vi "Image Acquiring Module.vi"(7 "Scan Status in":T1, 8 "Error in":errorcluster) -> (0 "Error Out":errorcluster)   [LabVIEW 2018]
uses:
  Controls/scan status.ctl
  Controls/FGV Actions.ctl
  Controls/Queue Manager Actions.ctl
  Controls/QueueNames.ctl
  Controls/MessagePacket.ctl
  Controls/Save Bline to Mem Control.ctl
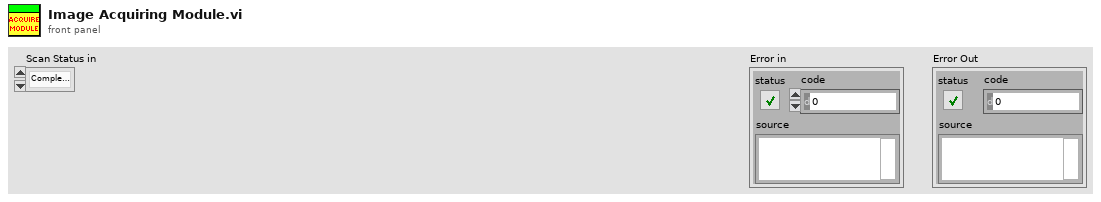
[diagram p1: front panel]
types:
  T1 = typedef "scan status.ctl" = enum16{"Complete Scan(ThorOCT)", "Complete Scan(PSOCT)", "Start(ThorOCT Spatial)", "Start(ThorOCT Spectral)", "Start(GPU FFT)", "Start(Alazar FFT)", "Scan(ThorOCT Spatial)", "Scan(ThorOCT Spectral)", "Scan(GPU FFT)", "Scan(Alazar FFT)", "Finish Scan(ThorOCT)", "Finish Scan(PSOCT)", "Scan(simulate)", "Start(ROI)"}
  T2 = typedef "FGV Actions.ctl" = enum16{"Init", "Set", "Get", "Clear"}
  T3 = typedef "System Parameters.ctl" = cluster{"Optical Parameters":T4, "Vibratome":T5, "Table Stages":T6, "Imaging Parameter":T9, "Galvo HW Parameters":cluster{"Analog Out Channel":tag, "Min Voltage":dbl, "Max Voltage":dbl, "Pixel Clock Source":tag, "Sample Rate":dbl, "Line Clock Out Ch":tag}, "Alazar parameters":T11, "Mosaic Paramter":cluster{"X Axis":cluster{"Start [mm]":dbl, "Steps [pts]":dbl, "End [mm]":dbl}, "Y Axis":cluster{"Start [mm]":dbl, "Steps [pts]":dbl, "End [mm]":dbl}, "Scan Pattern":enum16{"Uni-directional", "Bi-Directional", "Spiral Out", "Spiral In"}, "Overlap Options":cluster{"Overlap Type":enum16{"No Overlap", "X Only", "Y Only", "X and Y"}, "Percent Overlap":u8, "Justify":enum16{"Start", "Center", "End"}}}, "Manual Controls":T18, "Vibratome Axis":T21}
  T4 = typedef "Optical Parameters.ctl" = cluster{"Obj. Focal Length [mm]":dbl, "Scan Lens EFL[mm]":dbl, "Tube Lens EFL[mm]":dbl, "Galvo V Range (+/-)":dbl, "Galvo Max Half Angle [Deg]":dbl, "Max Galvo Range[%]":dbl}
  T5 = typedef "Vibratome Parameters.ctl" = cluster{"Z Bottom [mm]":dbl, "Pre Cut Dwell [s]":dbl, "Blade Frequency [RPM]":u16, "Slice Speed [mm/s]":dbl, "Post Cut Dwell [s]":dbl, "Ramp Time [s]":dbl, "Start X [mm]":dbl, "Start Y [mm]":dbl, "Slice Length [mm]":dbl, "Slice Axis":enum16{"X Axis", "Y Axis", "Z Axis"}, "Controller VISA Ref":refnum<visa-resource-name>, "Blade Frequency [Hz]":u16, "Analog Out Channel":tag, "Pixel Clock Source":tag}
  T6 = typedef "Translation Stage Parameters.ctl" = cluster{"X Stage":T7, "Y Stage":T7, "Z Stage":T7}
  T7 = typedef "Translation Stage Cluster.ctl" = cluster{"Position":dbl, "Is.Enabled?":bool, "Is.Connected?":bool, "Device SN":string, "AccelerationMaximum":dbl, "VelocityMaximum":dbl, "Acceleration":dbl, "Velocity":dbl, "waitTimeout (ms)":i32, "Model":T8, "Is.Homed?":bool}
  T8 = typedef "Translation Stage Types.ctl" = enum16{"None", "Thorlabs LTS", "Thorlabs MLJ"}
  T9 = typedef "Imaging Parameters.ctl" = cluster{"Raster Scan Direction":T10, "Pixel Dwell Time [Clock Cycles]":u16, "Flyback Time [Clock Cycles]":u16, "XY Center [um]":cluster{"X":dbl, "Y":dbl}, "Pixel Step Size [um] X":dbl, "XY Image Size":enum16{"32 x 32", "64 x 64", "128 x 128", "256 x 256", "512 x 512", "1024 x 1024", "2048 x 2048"}, "Custom":bool, "Custom Size":cluster{"X":u16, "Y":u16}, "Line Averages":u8, "Pixel Step Size [um] Y":dbl}
  T10 = typedef "Scan Direction.ctl" = enum16{"Uni Directional", "Bi Directional", "None"}
  T11 = typedef "Alazar parameters.ctl" = cluster{"Trigger Settings":cluster{"General Trigger Settings":T12, "Trigger Engine 1":T13, "Trigger Engine 2":T13}, "Device ID":T14, "Ch A Input Control":T15, "Ch B Input Control":T15, "Acq Settings":T16, "Capture Clock":T17}
  T12 = typedef "General Trigger Settings.ctl" = cluster{"Trigger Operation":u32, "Coupling ID":u32, "Range ID":u32, "Delay":u32, "Timeout Ticks":u32, "Mode":u32, "Parameter":u32}
  T13 = typedef "Trigger Engine Controls.ctl" = cluster{"Trigger Engine":u32, "Source":u32, "Slope":u32, "Level":u32}
  T14 = typedef "Alazar Device ID.ctl" = cluster{"System ID":u32, "Board ID":u32}
  T15 = typedef "Channel Input Controls.ctl" = cluster{"Channel":u8, "Coupling":u32, "Range":u32, "Impedance":u32}
  T16 = typedef "Alazar Acquisition Settings.ctl" = cluster{"Record Length":u32, "Offset":u32, "Records Per Buffer":u32, "Records Count (Records/Acq)":u32, "Window Type":u32, "Footer":u32, "Samples per record":u32, "Output Format":u32}
  T17 = typedef "Clock Controls.ctl" = cluster{"Sample Rate":u32, "Decimation":u32, "Source":u32, "Edge":u32}
  T18 = typedef "Manual Controls.ctl" = cluster{"Z0":dbl, "First image height":dbl, "Data Path":path, "Save parameters":T19, "Center Galvos":bool, "Acquisition mode":T20, "PSOCT Channel":u32, "Save":bool, "AIP rotation angle":dbl, "Scan Parameters":cluster{"# Scan":cluster{"#Ascan":i32, "#Bscan":i32}, "# Rpt":cluster{"#ARpt":i32, "#BRpt":i32}, "Aline Rate":u16, "# Extra":cluster{"# ARpt_extra":i32, "#Brtn_extra":i32}}, "ROI Parameters":cluster{"ROI (mm)":cluster{"X (mm)":dbl, "Y (mm)":dbl}, "Shift (mm)":cluster{"Xshift (mm)":sgl, "Yshift (mm)":sgl}}, "Objective":u16, "auto adjust focus":bool, "ret ds":bool, "Pause?":bool}
  T19 = typedef "FFT parameters.ctl" = cluster{"start pixel":i32, "#pixels to save":i32}
  T20 = typedef "FFT mode.ctl" = enum16{"ThorOCT B line", "ThorOCT Spectral", "ThorOCT FFT", "Alazar B line", "Alazar FFT", "GPU FFT", "Alazar Spectral", "Simulation", "auto adjust focus"}
  T21 = typedef "Vibratome Param.ctl" = cluster{"Start [mm](first cut height)":dbl, "slice thickness[um]":dbl, "#slice":u16, "slice thick2[um]":dbl, "#thin slices":u16, "image thickness(um)":dbl, "#images":u16, "image depth2":dbl, "#image depth2":u16}
  T22 = enum16{"Init", "Configure", "Configure Data", "Generate Scan Pattern", "Start Acquire Raw", "Start Acquire Data", "Acquire RAW", "Acquire Data", "Stop Acquire", "Uninit"}
  T23 = typedef "Save Bline to Mem Control.ctl" = enum16{"Output data", "Save(ThorOCT)", "Save(PSOCT)", "FFT and Save", "Uninit", "PSOCT Spectral buffer Set", "PSOCT Spatial buffer Set", "PSOCT Spectral buffer Init", "PSOCT Spatial buffer Init", "ThorOCT Spectral buffer Init", "ThorOCT Spatial buffer Init", "ThorOCT Spectral buffer Set", "ThorOCT Spatial buffer Set", "ThorOCT Spectral Save", "Alazar Spectral Save"}
  T24 = typedef "MessagePacket.ctl" = cluster{"Message":string, "Parameter":variant}
  T25 = typedef "QueueNames.ctl" = enum16{"Main GUI", "Main Scan Processor", "Main Processing", "Main Saving", "Main Display", "Main Table Stage GUI", "Main Table Stage Proc.", "Scan Engine", "Vibratome GUI", "Vibratome Processor", "Slice Engine"}
  T26 = typedef "Queue Manager Actions.ctl" = enum16{"Init", "Enqueue", "Enqueue All", "Preview Queue", "Dequeue", "Get Status", "Flush Queue", "Flush All Queues", "Release All Queues", "Release Queue", "Enqueue at Opposite End"}
  T27 = cluster{"# Scan":cluster{"#Ascan":i32, "#Bscan":i32}, "# Rpt":cluster{"#ARpt":i32, "#BRpt":i32}, "Aline Rate":u16, "# Extra":cluster{"# ARpt_extra":i32, "#Brtn_extra":i32}}
  T28 = cluster{"ROI (mm)":cluster{"X (mm)":dbl, "Y (mm)":dbl}, "Shift (mm)":cluster{"Xshift (mm)":sgl, "Yshift (mm)":sgl}}
  T29 = typedef "ScanType.ctl" = enum16{"Single Frame", "Continuous Frame", "ROI Line", "Vibratome", "Mosaic", "Mosaic + Slice"}
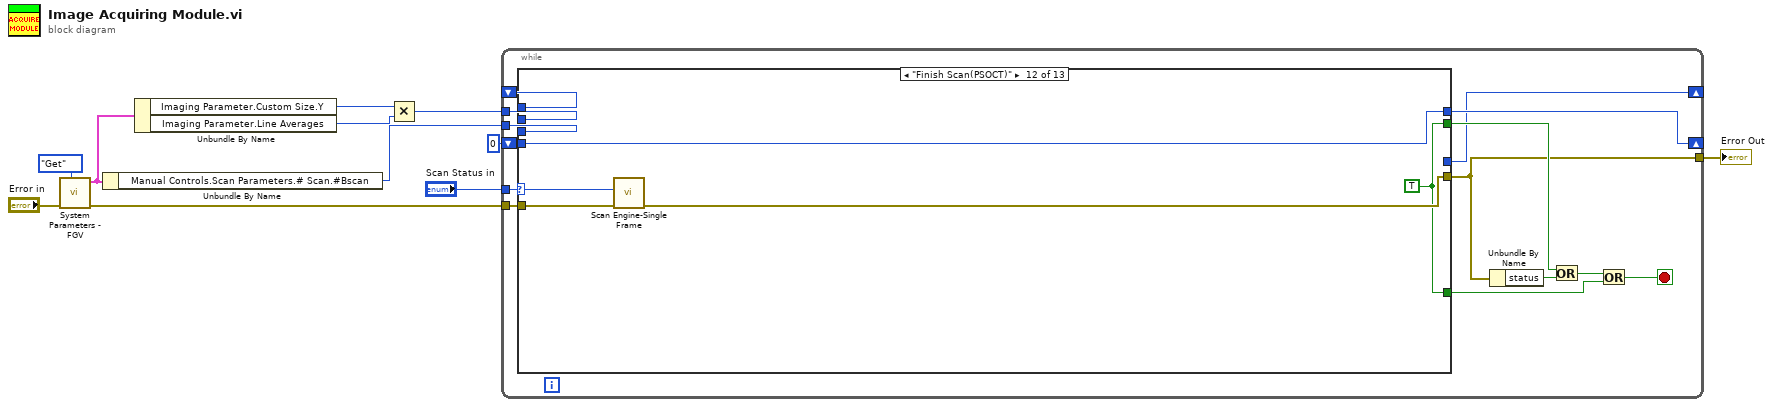
[diagram p0: block diagram]
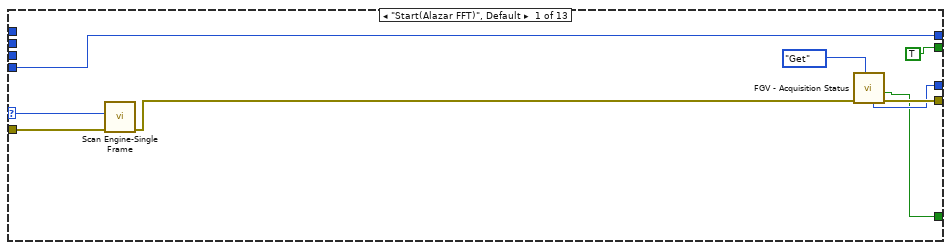
[diagram p2: hidden frame]
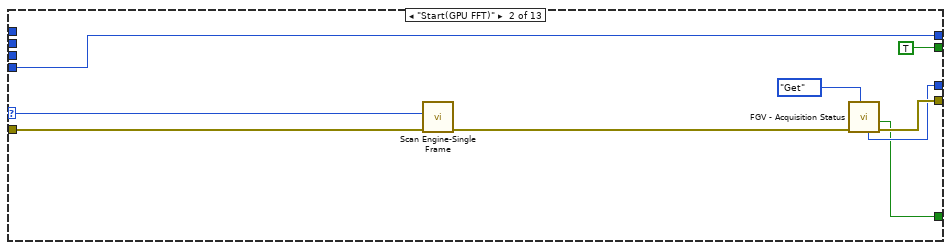
[diagram p3: hidden frame]
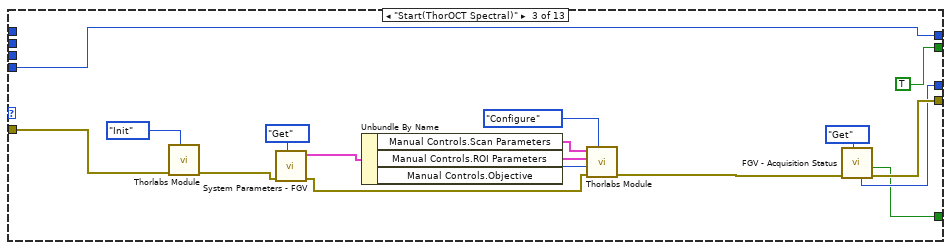
[diagram p4: hidden frame]
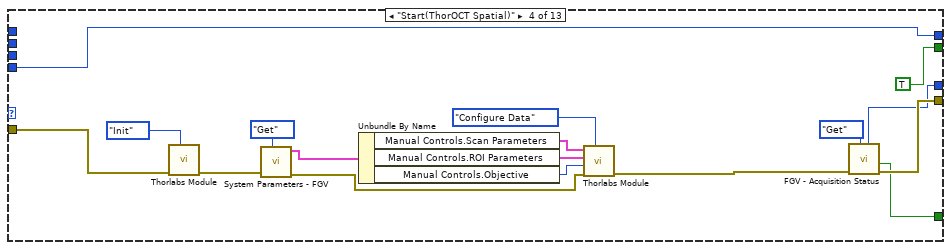
[diagram p5: hidden frame]
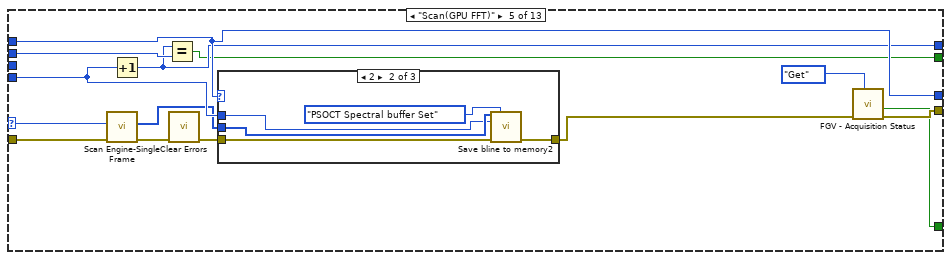
[diagram p6: hidden frame]
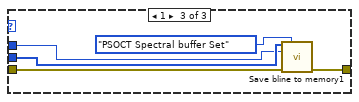
[diagram p8: hidden frame]
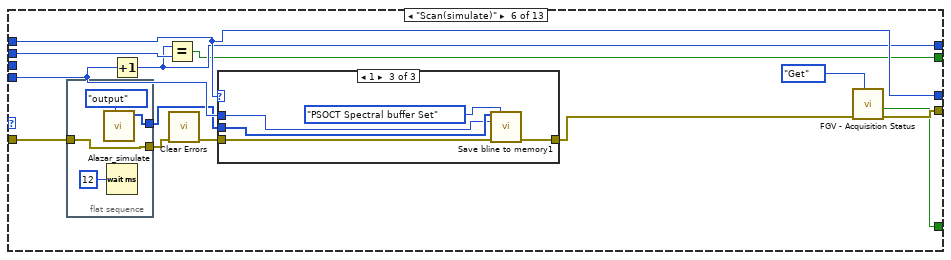
[diagram p9: hidden frame]
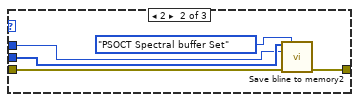
[diagram p11: hidden frame]
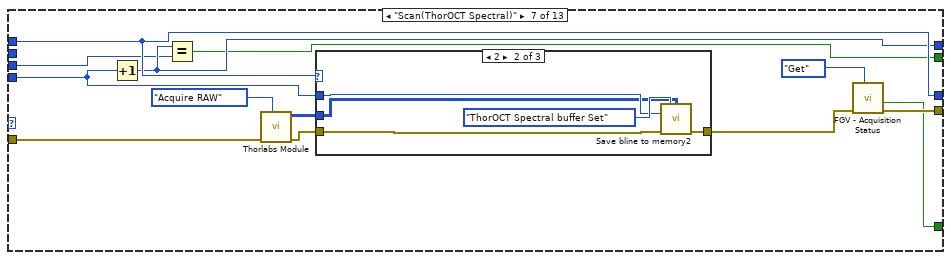
[diagram p12: hidden frame]
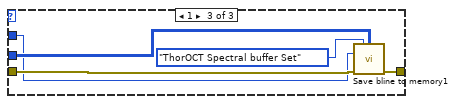
[diagram p14: hidden frame]
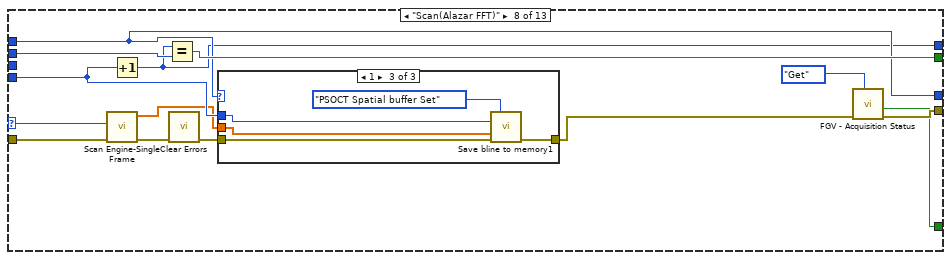
[diagram p15: hidden frame]
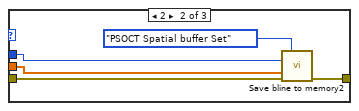
[diagram p17: hidden frame]
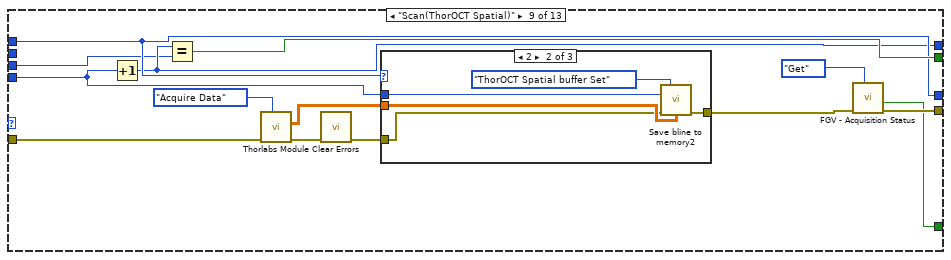
[diagram p18: hidden frame]
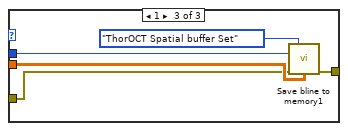
[diagram p20: hidden frame]
diagram:
  n1 = call "System Parameters - FGV.vi"("Actions"=FGV_Actions."Get", "Error In"="Error in") -> ("Error Out"=w2:errorcluster, "System Parameters [Out]"=w3:T3)  [unwired: 8 in]
  n2 = Unbundle By Name(w3) -> ("Manual Controls.Scan Parameters.# Scan.#Bscan"=w5:i32)
  n3 = Unbundle By Name(w3) -> ("Imaging Parameter.Custom Size.Y"=w8:u16, "Imaging Parameter.Line Averages"=w7:u8)
  n4 = Multiply(x=w8, y=w7) -> (x*y=w6:u16)
  n5 = while {
    tunnel: w2 -> [w23]
    tunnel: "Scan Status in" -> [w25]
    shift-right: [w24] -> _
    shift-left: u32 0 ("bline count") -> [w21]
    tunnel: w6 -> [w18]
    shift-right: [w16] -> _
    shift-left: _ -> [w17]
    tunnel: [w15] -> w9
    tunnel: w5 -> [w12]
    stop <- w19 stop-if-true
    n6 = case shown="\"Finish Scan(PSOCT)\"" w25 {
      selector: w25 -> [w31 w41 _ _ w85 _ _ w167 _ _ _ w246 _]
      tunnel: w23 -> [w34 w43 w54 w71 w86 w104 w135 w168 w184 w213 w226 w249 w252]
      tunnel: [w28 w37 w57 w74 w81 w108 w137 w159 w187 w208 w230 w247 w250] -> w15
      tunnel: [TRUE TRUE TRUE TRUE w87 w111 w140 w164 w192 TRUE ("task done?") TRUE ("task done?") w245 w254] -> w22
      tunnel: w21 -> [w32 w42 w60 w77 w88 w112 w141 w166 w193 _ _ w248 w255]
      tunnel: [w32 w42 w60 w77 w89 w113 w142 w162 w190 _ _ w248 w255] -> w24
      tunnel: w18 -> [_ _ _ _ w90 w114 _ w165 _ _ _ _ _]
      tunnel: w17 -> [_ _ _ _ w91 w115 w143 w163 w191 _ w223 _ _]
      tunnel: [w27 w36 w56 w73 w91 w115 w143 w163 w191 _ w222 _ _] -> w16
      tunnel: [w26 w35 w55 w72 w80 w107 w136 w158 w186 w206 w228 w245 w254] -> w13
      tunnel: w12 -> [_ _ _ _ _ _ w134 _ w183 _ _ _ _]
      frame "Start(Alazar FFT)", Default {
        n7 = call "Scan Engine-Single Frame.vi"("Error in"=w34, "Scan Status in"=w31) -> ("Error Out"=w29:errorcluster)  [unwired: 7 in, 2 out]
        n8 = call "FGV - Acquisition Status.vi"("Actions"=FGV_Actions."Get", "Error In"=w29) -> ("Error Out"=w28:errorcluster, "Quit status out"=w26:bool, "mem loc out"=w27:i32)  [unwired: 6 in, 1 out]
      }
      frame "Start(GPU FFT)" {
        n9 = call "Scan Engine-Single Frame.vi"("Error in"=w43, "Scan Status in"=w41) -> ("Error Out"=w38:errorcluster)  [unwired: 7 in, 2 out]
        n10 = call "FGV - Acquisition Status.vi"("Actions"=FGV_Actions."Get", "Error In"=w38) -> ("Error Out"=w37:errorcluster, "Quit status out"=w35:bool, "mem loc out"=w36:i32)  [unwired: 6 in, 1 out]
      }
      frame "Start(ThorOCT Spectral)" {
        n11 = call "Thorlabs Module.vi"("Actions"=T22."Init", "error in"=w54) -> ("error out"=w46:errorcluster)  [unwired: 6 in, 3 out]
        n12 = call "System Parameters - FGV.vi"("Actions"=FGV_Actions."Get", "Error In"=w46) -> ("Error Out"=w45:errorcluster, "System Parameters [Out]"=w44:T3)  [unwired: 8 in]
        n13 = Unbundle By Name(w44) -> ("Manual Controls.Scan Parameters"=w51:T27, "Manual Controls.ROI Parameters"=w49:T28, "Manual Controls.Objective"=w50:u16)
        n14 = call "Thorlabs Module.vi"("Actions"=T22."Configure", "error in"=w45, "Objective"=w50, "ROI Parameters"=w49, "Scan Parameters"=w51) -> ("error out"=w48:errorcluster)  [unwired: 3 in, 3 out]
        n15 = call "FGV - Acquisition Status.vi"("Actions"=FGV_Actions."Get", "Error In"=w48) -> ("Error Out"=w57:errorcluster, "Quit status out"=w55:bool, "mem loc out"=w56:i32)  [unwired: 6 in, 1 out]
      }
      frame "Start(ThorOCT Spatial)" {
        n16 = call "Thorlabs Module.vi"("Actions"=T22."Init", "error in"=w71) -> ("error out"=w63:errorcluster)  [unwired: 6 in, 3 out]
        n17 = call "System Parameters - FGV.vi"("Actions"=FGV_Actions."Get", "Error In"=w63) -> ("Error Out"=w62:errorcluster, "System Parameters [Out]"=w61:T3)  [unwired: 8 in]
        n18 = Unbundle By Name(w61) -> ("Manual Controls.Scan Parameters"=w68:T27, "Manual Controls.ROI Parameters"=w66:T28, "Manual Controls.Objective"=w67:u16)
        n19 = call "Thorlabs Module.vi"("Actions"=T22."Configure Data", "error in"=w62, "Objective"=w67, "ROI Parameters"=w66, "Scan Parameters"=w68) -> ("error out"=w65:errorcluster)  [unwired: 3 in, 3 out]
        n20 = call "FGV - Acquisition Status.vi"("Actions"=FGV_Actions."Get", "Error In"=w65) -> ("Error Out"=w74:errorcluster, "Quit status out"=w72:bool, "mem loc out"=w73:i32)  [unwired: 6 in, 1 out]
      }
      frame "Scan(GPU FFT)" {
        n21 = call "Scan Engine-Single Frame.vi"("Error in"=w86, "Scan Status in"=w85) -> ("Error Out"=w79:errorcluster, "Buffer"=w84:u16[])  [unwired: 7 in, 1 out]
        n22 = Increment(x=w88) -> (x+1=w89:u32)
        n23 = Equal?(x=w89, y=w90) -> (x = y?=w87:bool)
        n24 = call <vilib>:"Clear Errors.vi"("error in (no error)"=w79) -> ("error out"=w78:errorcluster)  [unwired: 5 in, 1 out]
        n25 = case shown="2" w91 {
          tunnel: w78 -> [w92 w97 w102]
          tunnel: [w92 w96 w101] -> w82
          tunnel: w88 -> [_ w93 w99]
          tunnel: w84 -> [_ w94 w100]
          frame 0, Default {
          }
          frame 2 {
            n26 = call "Save bline to memory2.vi"("PSOCTSpectral Bline"=w94, "action"=Save_Bline_to_Mem_Control."PSOCT Spectral buffer Set", "index (row)"=w93, "error in"=w97) -> ("error out"=w96:errorcluster)  [unwired: 11 in]
          }
          frame 1 {
            n27 = call "Save bline to memory1.vi"("PSOCTSpectral Bline"=w100, "action"=Save_Bline_to_Mem_Control."PSOCT Spectral buffer Set", "index (row)"=w99, "error in"=w102) -> ("error out"=w101:errorcluster)  [unwired: 11 in]
          }
        }
        n28 = call "FGV - Acquisition Status.vi"("Actions"=FGV_Actions."Get", "Error In"=w82) -> ("Error Out"=w81:errorcluster, "Quit status out"=w80:bool)  [unwired: 6 in, 2 out]
      }
      frame "Scan(simulate)" {
        n29 = flat-sequence {
          tunnel: [w119] -> w105
          tunnel: w104 -> [w117]
          tunnel: [w117] -> w103
          frame #0 {
            n30 = call "Alazar_simulate.vi"("Enum"=enum16{"init", "output"}."output") -> ("Array"=w119:u16[])  [unwired: 10 in]
            n31 = Wait (ms)(milliseconds to wait=u32 12) -> ()  [unwired: 1 out]
          }
        }
        n32 = Increment(x=w112) -> (x+1=w113:u32)
        n33 = Equal?(x=w113, y=w114) -> (x = y?=w111:bool)
        n34 = call <vilib>:"Clear Errors.vi"("error in (no error)"=w103) -> ("error out"=w106:errorcluster)  [unwired: 5 in, 1 out]
        n35 = case shown="1" w115 {
          tunnel: w106 -> [w120 w125 w130]
          tunnel: [w120 w124 w129] -> w109
          tunnel: w112 -> [_ w121 w127]
          tunnel: w105 -> [_ w122 w128]
          frame 0, Default {
          }
          frame 2 {
            n36 = call "Save bline to memory2.vi"("PSOCTSpectral Bline"=w122, "action"=Save_Bline_to_Mem_Control."PSOCT Spectral buffer Set", "index (row)"=w121, "error in"=w125) -> ("error out"=w124:errorcluster)  [unwired: 11 in]
          }
          frame 1 {
            n37 = call "Save bline to memory1.vi"("PSOCTSpectral Bline"=w128, "action"=Save_Bline_to_Mem_Control."PSOCT Spectral buffer Set", "index (row)"=w127, "error in"=w130) -> ("error out"=w129:errorcluster)  [unwired: 11 in]
          }
        }
        n38 = call "FGV - Acquisition Status.vi"("Actions"=FGV_Actions."Get", "Error In"=w109) -> ("Error Out"=w108:errorcluster, "Quit status out"=w107:bool)  [unwired: 6 in, 2 out]
      }
      frame "Scan(ThorOCT Spectral)" {
        n39 = Increment(x=w141) -> (x+1=w142:u32)
        n40 = Equal?(x=w142, y=w134) -> (x = y?=w140:bool)
        n41 = call "Thorlabs Module.vi"("Actions"=T22."Acquire RAW", "error in"=w135) -> ("error out"=w132:errorcluster, "Raw Data Out"=w131:u16[][])  [unwired: 6 in, 2 out]
        n42 = case shown="2" w143 {
          tunnel: w132 -> [w144 w149 w154]
          tunnel: [w144 w148 w153] -> w138
          tunnel: w141 -> [_ w146 w151]
          tunnel: w131 -> [_ w145 w152]
          frame 0, Default {
          }
          frame 2 {
            n43 = call "Save bline to memory2.vi"("action"=Save_Bline_to_Mem_Control."ThorOCT Spectral buffer Set", "ThorOCT Spectral Bline"=w145, "index (row)"=w146, "error in"=w149) -> ("error out"=w148:errorcluster)  [unwired: 11 in]
          }
          frame 1 {
            n44 = call "Save bline to memory1.vi"("action"=Save_Bline_to_Mem_Control."ThorOCT Spectral buffer Set", "ThorOCT Spectral Bline"=w152, "index (row)"=w151, "error in"=w154) -> ("error out"=w153:errorcluster)  [unwired: 11 in]
          }
        }
        n45 = call "FGV - Acquisition Status.vi"("Actions"=FGV_Actions."Get", "Error In"=w138) -> ("Error Out"=w137:errorcluster, "Quit status out"=w136:bool)  [unwired: 6 in, 2 out]
      }
      frame "Scan(Alazar FFT)" {
        n46 = call "Scan Engine-Single Frame.vi"("Error in"=w168, "Scan Status in"=w167) -> ("Error Out"=w156:errorcluster, "FFT Buffer"=w155:sgl[])  [unwired: 7 in, 1 out]
        n47 = Increment(x=w166) -> (x+1=w162:u32)
        n48 = Equal?(x=w162, y=w165) -> (x = y?=w164:bool)
        n49 = call <vilib>:"Clear Errors.vi"("error in (no error)"=w156) -> ("error out"=w157:errorcluster)  [unwired: 5 in, 1 out]
        n50 = case shown="1" w163 {
          tunnel: w157 -> [w169 w171 w176]
          tunnel: [w169 w170 w175] -> w160
          tunnel: w166 -> [_ w174 w178]
          tunnel: w155 -> [_ w173 w179]
          frame 0, Default {
          }
          frame 2 {
            n51 = call "Save bline to memory2.vi"("action"=Save_Bline_to_Mem_Control."PSOCT Spatial buffer Set", "index (row)"=w174, "PSOCT Spatial Bline"=w173, "error in"=w171) -> ("error out"=w170:errorcluster)  [unwired: 11 in]
          }
          frame 1 {
            n52 = call "Save bline to memory1.vi"("action"=Save_Bline_to_Mem_Control."PSOCT Spatial buffer Set", "index (row)"=w178, "PSOCT Spatial Bline"=w179, "error in"=w176) -> ("error out"=w175:errorcluster)  [unwired: 11 in]
          }
        }
        n53 = call "FGV - Acquisition Status.vi"("Actions"=FGV_Actions."Get", "Error In"=w160) -> ("Error Out"=w159:errorcluster, "Quit status out"=w158:bool)  [unwired: 6 in, 2 out]
      }
      frame "Scan(ThorOCT Spatial)" {
        n54 = Increment(x=w193) -> (x+1=w190:u32)
        n55 = Equal?(x=w190, y=w183) -> (x = y?=w192:bool)
        n56 = call "Thorlabs Module.vi"("Actions"=T22."Acquire Data", "error in"=w184) -> ("error out"=w181:errorcluster, "Data Out"=w180:sgl[][])  [unwired: 6 in, 2 out]
        n57 = call <vilib>:"Clear Errors.vi"("error in (no error)"=w181) -> ("error out"=w185:errorcluster)  [unwired: 5 in, 1 out]
        n58 = case shown="2" w191 {
          tunnel: w185 -> [w194 w196 w201]
          tunnel: [w194 w195 w200] -> w188
          tunnel: w193 -> [_ w199 w204]
          tunnel: w180 -> [_ w197 w202]
          frame 0, Default {
          }
          frame 2 {
            n59 = call "Save bline to memory2.vi"("action"=Save_Bline_to_Mem_Control."ThorOCT Spatial buffer Set", "index (row)"=w199, "error in"=w196, "ThorOCT Spatial Bline"=w197) -> ("error out"=w195:errorcluster)  [unwired: 11 in]
          }
          frame 1 {
            n60 = call "Save bline to memory1.vi"("action"=Save_Bline_to_Mem_Control."ThorOCT Spatial buffer Set", "index (row)"=w204, "error in"=w201, "ThorOCT Spatial Bline"=w202) -> ("error out"=w200:errorcluster)  [unwired: 11 in]
          }
        }
        n61 = call "FGV - Acquisition Status.vi"("Actions"=FGV_Actions."Get", "Error In"=w188) -> ("Error Out"=w187:errorcluster, "Quit status out"=w186:bool)  [unwired: 6 in, 2 out]
      }
      frame "Complete Scan(PSOCT)" {
        n62 = call "FGV - Acquisition Status.vi"("Actions"=FGV_Actions."Get", "Error In"=w213) -> ("Error Out"=w210:errorcluster, "Quit status out"=w206:bool, "Scan Type [Out]"=w205:T29, "mem loc out"=w212:i32)  [unwired: 6 in]
        n63 = case shown="1" w212 {
          tunnel: [1 2] -> w207
          frame 2, Default {
          }
          frame 1 {
          }
        }
        n64 = call "FGV - Acquisition Status.vi"("mem loc"=w207, "Actions"=FGV_Actions."Set", "Error In"=w210, "Quit status"=w206, "Scan Type [In]"=w205) -> ("Error Out"=w209:errorcluster)  [unwired: 3 in, 3 out]
        n65 = Build Array(T24 {"Message"="Process", "Parameter"=variant} ("Message Packet Array")) -> (w216:T24[])
        n66 = call "Queue Manager.vi"("Queue Name"=QueueNames."Main Processing", "Action"=Queue_Manager_Actions."Enqueue", "Error In"=w209, "Message Packet Array"=w216) -> ("Error Out"=w208:errorcluster)  [unwired: 3 in, 4 out]
      }
      frame "Complete Scan(ThorOCT)" {
        n67 = case shown="2, Default" w223 {
          tunnel: [1 2] -> w222
          frame 2, Default {
          }
          frame 1 {
          }
        }
        n68 = call "Thorlabs Module.vi"("Actions"=T22."Stop Acquire", "error in"=w226) -> ("error out"=w225:errorcluster)  [unwired: 6 in, 3 out]
        n69 = call "FGV - Acquisition Status.vi"("Actions"=FGV_Actions."Get", "Error In"=w225) -> ("Error Out"=w232:errorcluster, "Quit status out"=w228:bool, "Scan Type [Out]"=w227:T29, "mem loc out"=w234:i32)  [unwired: 6 in]
        n70 = case shown="2, Default" w234 {
          tunnel: [1 2] -> w229
          frame 2, Default {
          }
          frame 1 {
          }
        }
        n71 = call "FGV - Acquisition Status.vi"("mem loc"=w229, "Actions"=FGV_Actions."Set", "Error In"=w232, "Quit status"=w228, "Scan Type [In]"=w227) -> ("Error Out"=w231:errorcluster)  [unwired: 3 in, 3 out]
        n72 = Build Array(T24 {"Message"="Process", "Parameter"=variant} ("Message Packet Array")) -> (w237:T24[])
        n73 = call "Queue Manager.vi"("Queue Name"=QueueNames."Main Processing", "Action"=Queue_Manager_Actions."Enqueue", "Error In"=w231, "Message Packet Array"=w237) -> ("Error Out"=w230:errorcluster)  [unwired: 3 in, 4 out]
      }
      frame "Finish Scan(PSOCT)" {
        w245 = TRUE ("task done?")
        n74 = call "Scan Engine-Single Frame.vi"("Error in"=w249, "Scan Status in"=w246) -> ("Error Out"=w247:errorcluster)  [unwired: 7 in, 2 out]
      }
      frame "Finish Scan(ThorOCT)" {
        w254 = TRUE ("task done?")
        n75 = call "Thorlabs Module.vi"("Actions"=T22."Uninit", "error in"=w252) -> ("error out"=w251:errorcluster)  [unwired: 6 in, 3 out]
        n76 = call <vilib>:"Clear Errors.vi"("error in (no error)"=w251) -> ("error out"=w250:errorcluster)  [unwired: 5 in, 1 out]
      }
    }
    n77 = Unbundle By Name(w15) -> ("status"=w14:bool)
    n78 = Or(x=w22, y=w14) -> (x .or. y?=w20:bool)
    n79 = Or(x=w20, y=w13) -> (x .or. y?=w19:bool)
  }
  "Error Out" <- w9
